vi "Data Change Process.vi"(8 "error in (no error)":errorcluster, 10 "data change":T1={"node ID"="", " value"=variant, "timestamp"=timestamp(0 s since 1904-01-01), "data type"=1, "status code"=0} {"data type" items=["Boolean"=1, "SByte"=2, "Byte"=3, "Int16"=4, "UInt16"=5, "Int32"=6, "UInt32"=7, "Int64"=8, "UInt64"=9, "Float"=10, "Double"=11, "String"=12, "DateTime"=13, "ByteString"=15, "Array of Boolean"=101, "Array of SByte"=102, "Array of Byte"=103, "Array of Int16"=104, "Array of UInt16"=105, "Array of Int32"=106, "Array of UInt32"=107, "Array of Int64"=108, "Array of UInt64"=109, "Array of Float"=110, "Array of Double"=111, "Array of String"=112, "Array of DateTime"=113, "Array of ByteString"=115, "Matrix of Boolean"=201, "Matrix of SByte"=202, "Matrix of Byte"=203, "Matrix of Int16"=204, "Matrix of UInt16"=205, "Matrix of Int32"=206, "Matrix of UInt32"=207, "Matrix of Int64"=208, "Matrix of UInt64"=209, "Matrix of Float"=210, "Matrix of Double"=211, "Matrix of String "=212, "Matrix of DateTime"=213, "Matrix of ByteString"=215]; "status code" items=["Good"=0, "Good_SubscriptionTransferred"=2949120, "Good_CompletesAsynchronously"=3014656, "Good_Overload"=3080192, "Good_Clamped"=3145728, "Good_LocalOverride"=9830400, "Good_EntryInserted"=10616832, "Good_EntryReplaced"=10682368, "Good_NoData"=10813440, "Good_MoreData"=10878976, "Good_CommunicationEvent"=10944512, "Good_ShutdownEvent"=11010048, "Good_CallAgain"=11075584, "Good_NonCriticalTimeout"=11141120, "Good_ResultsMayBeIncomplete"=12189696, "Good_DataIgnored"=14221312, "Uncertain"=1073741824, "Uncertain_ReferenceOutOfServer"=1080819712, "Uncertain_NoCommunicationLastUsableValue"=1083113472, "Uncertain_LastUsableValue"=1083179008, "Uncertain_SubstituteValue"=1083244544, "Uncertain_InitialValue"=1083310080, "Uncertain_SensorNotAccurate"=1083375616, "Uncertain_EngineeringUnitsExceeded"=1083441152, "Uncertain_SubNormal"=1083506688, "Uncertain_DataSubNormal"=1084489728, "Uncertain_ReferenceNotDeleted"=1086062592, "Uncertain_NotAllNodesAvailable"=1086324736, "Bad"=2147483648, "Bad_UnexpectedError"=2147549184, "Bad_InternalError"=2147614720, "Bad_OutOfMemory"=2147680256, "Bad_ResourceUnavailable"=2147745792, "Bad_CommunicationError"=2147811328, "Bad_EncodingError"=2147876864, "Bad_DecodingError"=2147942400, "Bad_EncodingLimitsExceeded"=2148007936, "Bad_UnknownResponse"=2148073472, "Bad_Timeout"=2148139008, "Bad_ServiceUnsupported"=2148204544, "Bad_Shutdown"=2148270080, "Bad_ServerNotConnected"=2148335616, "Bad_ServerHalted"=2148401152, "Bad_NothingToDo"=2148466688, "Bad_TooManyOperations"=2148532224, "Bad_DataTypeIdUnknown"=2148597760, "Bad_CertificateInvalid"=2148663296, "Bad_SecurityChecksFailed"=2148728832, "Bad_CertificateTimeInvalid"=2148794368, "Bad_CertificateIssuerTimeInvalid"=2148859904, "Bad_CertificateHostNameInvalid"=2148925440, "Bad_CertificateUriInvalid"=2148990976, "Bad_CertificateUseNotAllowed"=2149056512, "Bad_CertificateIssuerUseNotAllowed"=2149122048, "Bad_CertificateUntrusted"=2149187584, "Bad_CertificateRevocationUnknown"=2149253120, "Bad_CertificateIssuerRevocationUnknown"=2149318656, "Bad_CertificateRevoked"=2149384192, "Bad_CertificateIssuerRevoked"=2149449728, "Bad_UserAccessDenied"=2149515264, "Bad_IdentityTokenInvalid"=2149580800, "Bad_IdentityTokenRejected"=2149646336, "Bad_SecureChannelIdInvalid"=2149711872, "Bad_InvalidTimestamp"=2149777408, "Bad_NonceInvalid"=2149842944, "Bad_SessionIdInvalid"=2149908480, "Bad_SessionClosed"=2149974016, "Bad_SessionNotActivated"=2150039552, "Bad_SubscriptionIdInvalid"=2150105088, "Bad_RequestHeaderInvalid"=2150236160, "Bad_TimestampsToReturnInvalid"=2150301696, "Bad_RequestCancelledByClient"=2150367232, "Bad_NoCommunication"=2150694912, "Bad_WaitingForInitialData"=2150760448, "Bad_NodeIdInvalid"=2150825984, "Bad_NodeIdUnknown"=2150891520, "Bad_AttributeIdInvalid"=2150957056, "Bad_IndexRangeInvalid"=2151022592, "Bad_IndexRangeNoData"=2151088128, "Bad_DataEncodingInvalid"=2151153664, "Bad_DataEncodingUnsupported"=2151219200, "Bad_NotReadable"=2151284736, "Bad_NotWritable"=2151350272, "Bad_OutOfRange"=2151415808, "Bad_NotSupported"=2151481344, "Bad_NotFound"=2151546880, "Bad_ObjectDeleted"=2151612416, "Bad_NotImplemented"=2151677952, "Bad_MonitoringModeInvalid"=2151743488, "Bad_MonitoredItemIdInvalid"=2151809024, "Bad_MonitoredItemFilterInvalid"=2151874560, "Bad_MonitoredItemFilterUnsupported"=2151940096, "Bad_FilterNotAllowed"=2152005632, "Bad_StructureMissing"=2152071168, "Bad_EventFilterInvalid"=2152136704, "Bad_ContentFilterInvalid"=2152202240, "Bad_FilterOperandInvalid"=2152267776, "Bad_ContinuationPointInvalid"=2152333312, "Bad_NoContinuationPoints"=2152398848, "Bad_ReferenceTypeIdInvalid"=2152464384, "Bad_BrowseDirectionInvalid"=2152529920, "Bad_NodeNotInView"=2152595456, "Bad_ServerUriInvalid"=2152660992, "Bad_ServerNameMissing"=2152726528, "Bad_DiscoveryUrlMissing"=2152792064, "Bad_SempahoreFileMissing"=2152857600, "Bad_RequestTypeInvalid"=2152923136, "Bad_SecurityModeRejected"=2152988672, "Bad_SecurityPolicyRejected"=2153054208, "Bad_TooManySessions"=2153119744, "Bad_UserSignatureInvalid"=2153185280, "Bad_ApplicationSignatureInvalid"=2153250816, "Bad_NoValidCertificates"=2153316352, "Bad_RequestCancelledByRequest"=2153381888, "Bad_ParentNodeIdInvalid"=2153447424, "Bad_ReferenceNotAllowed"=2153512960, "Bad_NodeIdRejected"=2153578496, "Bad_NodeIdExists"=2153644032, "Bad_NodeClassInvalid"=2153709568, "Bad_BrowseNameInvalid"=2153775104, "Bad_BrowseNameDuplicated"=2153840640, "Bad_NodeAttributesInvalid"=2153906176, "Bad_TypeDefinitionInvalid"=2153971712, "Bad_SourceNodeIdInvalid"=2154037248, "Bad_TargetNodeIdInvalid"=2154102784, "Bad_DuplicateReferenceNotAllowed"=2154168320, "Bad_InvalidSelfReference"=2154233856, "Bad_ReferenceLocalOnly"=2154299392, "Bad_NoDeleteRights"=2154364928, "Bad_ServerIndexInvalid"=2154430464, "Bad_ViewIdUnknown"=2154496000, "Bad_TooManyMatches"=2154627072, "Bad_QueryTooComplex"=2154692608, "Bad_NoMatch"=2154758144, "Bad_MaxAgeInvalid"=2154823680, "Bad_HistoryOperationInvalid"=2154889216, "Bad_HistoryOperationUnsupported"=2154954752, "Bad_WriteNotSupported"=2155020288, "Bad_TypeMismatch"=2155085824, "Bad_MethodInvalid"=2155151360, "Bad_ArgumentsMissing"=2155216896, "Bad_TooManySubscriptions"=2155282432, "Bad_TooManyPublishRequests"=2155347968, "Bad_NoSubscription"=2155413504, "Bad_SequenceNumberUnknown"=2155479040, "Bad_MessageNotAvailable"=2155544576, "Bad_InsufficientClientProfile"=2155610112, "Bad_TcpServerTooBusy"=2155675648, "Bad_TcpMessageTypeInvalid"=2155741184, "Bad_TcpSecureChannelUnknown"=2155806720, "Bad_TcpMessageTooLarge"=2155872256, "Bad_TcpNotEnoughResources"=2155937792, "Bad_TcpInternalError"=2156003328, "Bad_TcpEndpointUrlInvalid"=2156068864, "Bad_RequestInterrupted"=2156134400, "Bad_RequestTimeout"=2156199936, "Bad_SecureChannelClosed"=2156265472, "Bad_SecureChannelTokenUnknown"=2156331008, "Bad_SequenceNumberInvalid"=2156396544, "Bad_ConfigurationError"=2156462080, "Bad_NotConnected"=2156527616, "Bad_DeviceFailure"=2156593152, "Bad_SensorFailure"=2156658688, "Bad_OutOfService"=2156724224, "Bad_DeadbandFilterInvalid"=2156789760, "Bad_RefreshInProgress"=2157379584, "Bad_ConditionAlreadyDisabled"=2157445120, "Bad_ConditionDisabled"=2157510656, "Bad_EventIdUnknown"=2157576192, "Bad_NoData"=2157641728, "Bad_DataLost"=2157772800, "Bad_DataUnavailable"=2157838336, "Bad_EntryExists"=2157903872, "Bad_NoEntryExists"=2157969408, "Bad_TimestampNotSupported"=2158034944, "Bad_InvalidArgument"=2158690304, "Bad_ConnectionRejected"=2158755840, "Bad_Disconnect"=2158821376, "Bad_ConnectionClosed"=2158886912, "Bad_InvalidState"=2158952448, "Bad_EndOfStream"=2159017984, "Bad_NoDataAvailable"=2159083520, "Bad_WaitingForResponse"=2159149056, "Bad_OperationAbandoned"=2159214592, "Bad_ExpectedStreamToBlock"=2159280128, "Bad_WouldBlock"=2159345664, "Bad_SyntaxError"=2159411200, "Bad_MaxConnectionsReached"=2159476736, "Bad_RequestTooLarge"=2159542272, "Bad_ResponseTooLarge"=2159607808, "Bad_EventNotAcknowledgeable"=2159738880, "Bad_InvalidTimestampArgument"=2159869952, "Bad_ProtocolVersionUnsupported"=2159935488, "Bad_StateNotActive"=2160001024, "Bad_FilterOperatorInvalid"=2160132096, "Bad_FilterOperatorUnsupported"=2160197632, "Bad_FilterOperandCountMismatch"=2160263168, "Bad_FilterElementInvalid"=2160328704, "Bad_FilterLiteralInvalid"=2160394240, "Bad_IdentityChangeNotSupported"=2160459776, "Bad_NotTypeDefinition"=2160590848, "Bad_ViewTimestampInvalid"=2160656384, "Bad_ViewParameterMismatch"=2160721920, "Bad_ViewVersionInvalid"=2160787456, "Bad_ConditionAlreadyEnabled"=2160852992, "Bad_DialogNotActive"=2160918528, "Bad_DialogResponseInvalid"=2160984064, "Bad_ConditionBranchAlreadyAcked"=2161049600, "Bad_ConditionBranchAlreadyConfirmed"=2161115136, "Bad_ConditionAlreadyShelved"=2161180672, "Bad_ConditionNotShelved"=2161246208, "Bad_ShelvingTimeOutOfRange"=2161311744, "Bad_AggregateListMismatch"=2161377280, "Bad_AggregateNotSupported"=2161442816, "Bad_AggregateInvalidInputs"=2161508352, "Bad_BoundNotFound"=2161573888, "Bad_BoundNotSupported"=2161639424, "Bad_AggregateConfigurationRejected"=2161770496, "Bad_TooManyMonitoredItems"=2161836032]}, 11 "Model in":refnum<class "Model.lvclass">) -> (0 "error out":errorcluster, 3 "Model out":refnum<class "Model.lvclass">)   [LabVIEW 2021, in "Model.lvlib" / "Model.lvclass"]
uses:
  Model.lvclass
  <vilib>/OPCUA/controls/Subscription Data Change.ctl
  <vilib>/OPCUA/controls/NodeId.ctl
  <vilib>/OPCUA/controls/Data Type.ctl
  <vilib>/OPCUA/controls/OPC UA StatusCode.ctl
  Model.lvclass/Model.ctl
  95c299c4-6619-4fcf-af27-bee369d36df4.vi
  <userlib>/John_Lib/AMC_FW/Send Local Message.vi
  <userlib>/John_Lib/AMC_FW/Create Single Message.vi
  <userlib>/John_Lib/AMC_FW/Update Message Routing Info.vi
  <userlib>/John_Lib/OPCUA/add NameSpace for single NoteID.vi
  <vilib>/OPCUA/client/internal/Read.vi
  <vilib>/OPCUA/client/internal/Read String.vi
  <userlib>/John_Lib/AMC_FW/String to Array.vi
  <vilib>/Utility/Data Type/Get Type Information.vi
  <userlib>/John_Lib/AMC_FW/Send Message.vi
  <userlib>/John_Lib/OPCUA/OPCUA.lvclass
  <vilib>/Utility/miscctls.llb/LVStringsAndValuesArrayTypeDef_U16.ctl
panel:
  out "x = y?":bool
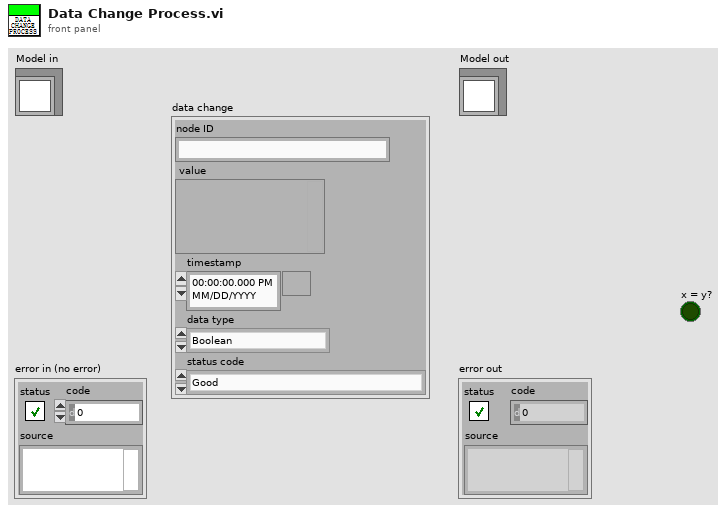
[diagram p1: front panel]
types:
  T1 = typedef "Subscription Data Change.ctl" = cluster{"node ID":T2, " value":variant, "timestamp":timestamp, "data type":T3, "status code":T4}
  T2 = typedef "NodeId.ctl" = string
  T3 = typedef "Data Type.ctl" = u16
  T4 = typedef "OPC UA StatusCode.ctl" = u32
  T5 = typedef "AMC_FW.lvlib/Queue.ctl" = cluster{"Q":T6, "Name":string}
  T6 = typedef "AMC_FW.lvlib/Message Queue.ctl" = refnum<queue>
  T7 = typedef "LVStringsAndValuesArrayTypeDef_U16.ctl" = cluster{"String":string, "Value":u16}[]
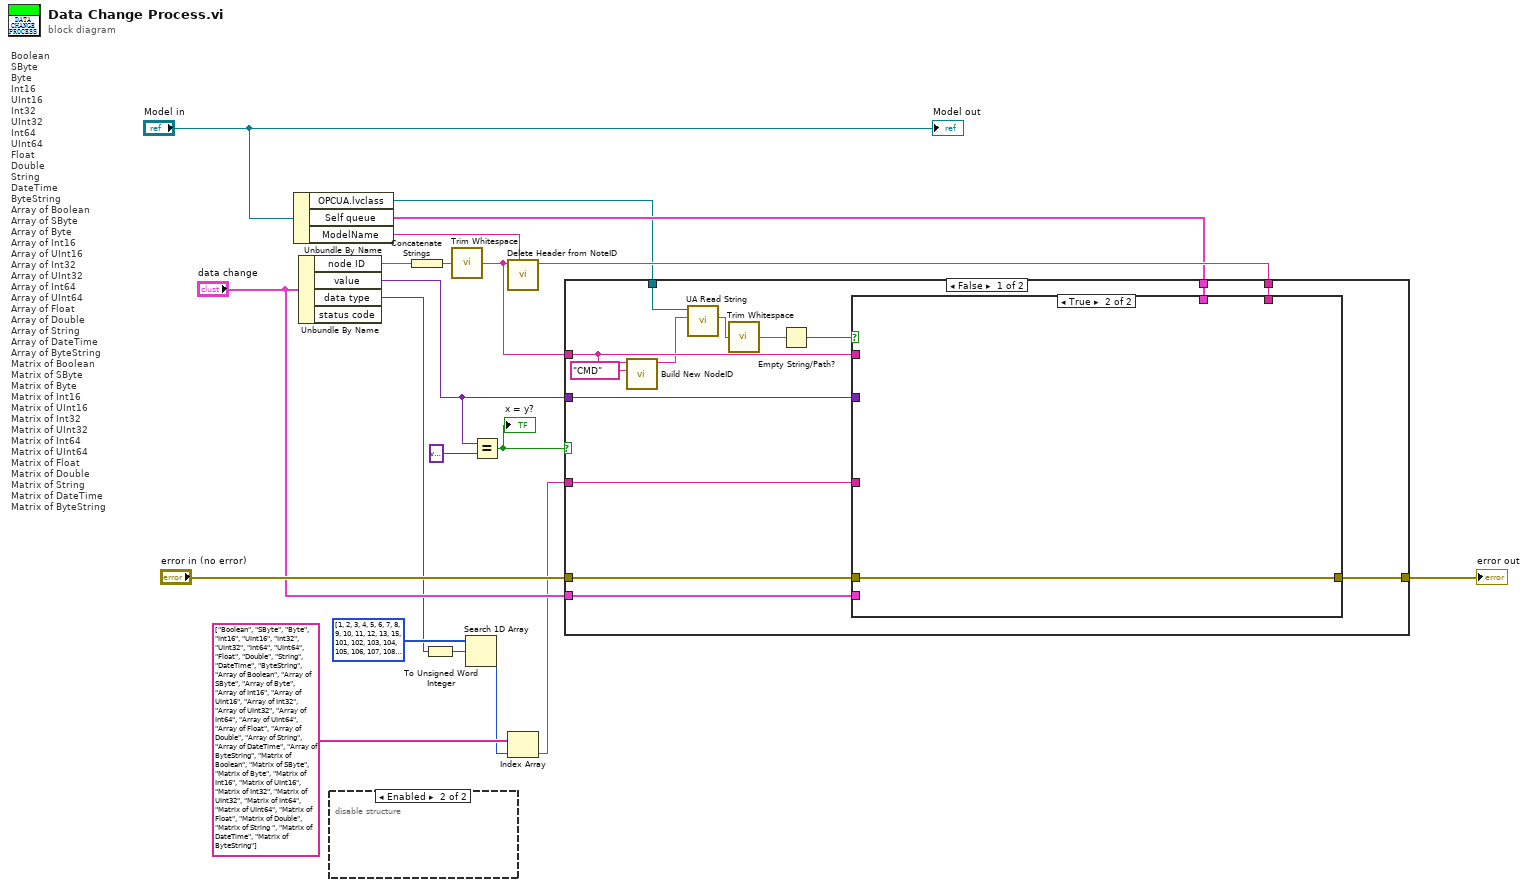
[diagram p0: block diagram]
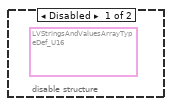
[diagram p2: hidden frame]
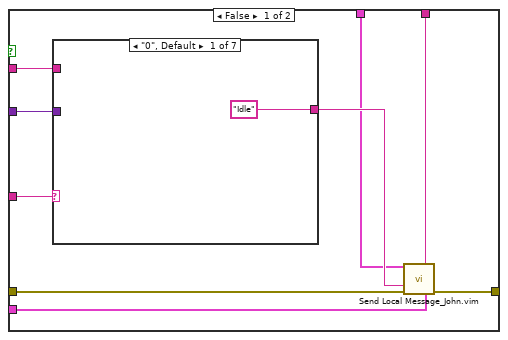
[diagram p3: hidden frame]
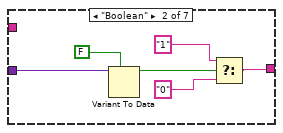
[diagram p4: hidden frame]
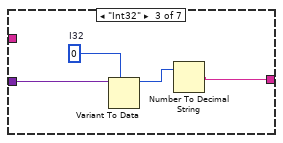
[diagram p5: hidden frame]
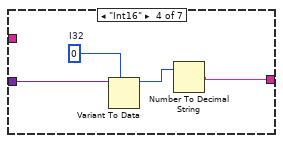
[diagram p6: hidden frame]
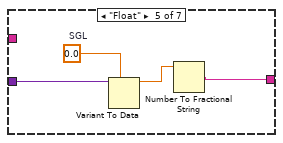
[diagram p7: hidden frame]
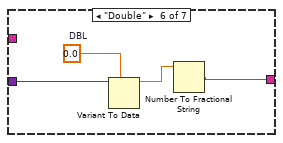
[diagram p8: hidden frame]
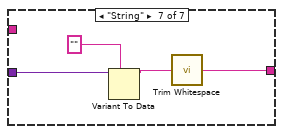
[diagram p9: hidden frame]
diagram:
  # "Boolean\nSByte\nByte\nInt16\nUInt16\nInt32\nUInt32\nInt64\nUInt64\nFloat\nDouble\nString\nDateTime\nByteString\nArray of Boolean\nArray of SByte\nArray of Byte\nArray of Int16\nArray of UInt16\nArray of Int32\nArray of UInt32\nArray of Int64\nArray of UInt64\nArray of Float\nArray of Double\nArray of String\nArray of DateTime\nArray of ByteString\nMatrix of Boolean\nMatrix of SByte\nMatrix of Byte\nMatrix of Int16\nMatrix of UInt16\nMatrix of Int32\nMatrix of UInt32\nMatrix of Int64\nMatrix of UInt64\nMatrix of Float\nMatrix of Double\nMatrix of String \nMatrix of DateTime\nMatrix of ByteString"
  n1 = Unbundle By Name("Model in") -> ("OPCUA.lvclass"=w1:refnum<class "OPCUA.lvclass">, "Self queue"=w14:T5, "ModelName"=w19:string)
  n2 = Unbundle By Name("data change") -> ("node ID"=w18:T2, "value"=w11:variant, "data type"=w6:T3)  [unwired: 1 out]
  n3 = disable-structure shown="Enabled" {
    frame Disabled {
      (unwired) T7 [{"String"="Boolean", "Value"=1}, {"String"="SByte", "Value"=2}, {"String"="Byte", "Value"=3}, {"String"="Int16", "Value"=4}, {"String"="UInt16", "Value"=5}, {"String"="Int32", "Value"=6}, {"String"="UInt32", "Value"=7}, {"String"="Int64", "Value"=8}, {"String"="UInt64", "Value"=9}, {"String"="Float", "Value"=10}, {"String"="Double", "Value"=11}, {"String"="String", "Value"=12}, {"String"="DateTime", "Value"=13}, {"String"="ByteString", "Value"=15}, {"String"="Array of Boolean", "Value"=101}, {"String"="Array of SByte", "Value"=102}, {"String"="Array of Byte", "Value"=103}, {"String"="Array of Int16", "Value"=104}, {"String"="Array of UInt16", "Value"=105}, {"String"="Array of Int32", "Value"=106}, {"String"="Array of UInt32", "Value"=107}, {"String"="Array of Int64", "Value"=108}, {"String"="Array of UInt64", "Value"=109}, {"String"="Array of Float", "Value"=110}, {"String"="Array of Double", "Value"=111}, {"String"="Array of String", "Value"=112}, {"String"="Array of DateTime", "Value"=113}, {"String"="Array of ByteString", "Value"=115}, {"String"="Matrix of Boolean", "Value"=201}, {"String"="Matrix of SByte", "Value"=202}, {"String"="Matrix of Byte", "Value"=203}, {"String"="Matrix of Int16", "Value"=204}, {"String"="Matrix of UInt16", "Value"=205}, {"String"="Matrix of Int32", "Value"=206}, {"String"="Matrix of UInt32", "Value"=207}, {"String"="Matrix of Int64", "Value"=208}, {"String"="Matrix of UInt64", "Value"=209}, {"String"="Matrix of Float", "Value"=210}, {"String"="Matrix of Double", "Value"=211}, {"String"="Matrix of String ", "Value"=212}, {"String"="Matrix of DateTime", "Value"=213}, {"String"="Matrix of ByteString", "Value"=215}] ("Strings And Values []")
    }
    frame Enabled {
    }
  }
  n4 = Concatenate Strings(w18) -> (w17:string)
  n5 = To Unsigned Word Integer(number=w6) -> (unsigned 16bit integer=w5:T3)
  n6 = call <vilib>:"Trim Whitespace.vi"("string"=w17) -> ("trimmed string"=w16:string)  [unwired: 1 in]
  n7 = Search 1D Array(1D array=u16[] [1, 2, 3, 4, 5, 6, 7, 8, 9, 10, 11, 12, 13, 15, 101, 102, 103, 104, 105, 106, 107, 108, 109, 110, 111, 112, 113, 115, 201, 202, 203, 204, 205, 206, 207, 208, 209, 210, 211, 212, 213, 215] ("Array 2"), element=w5) -> (index of element=w3:i32)  [unwired: 1 in]
  n8 = Equal?(x=w11, y=variant ("variant")) -> (x = y?=w9:bool)
  "x = y?" <- w9
  n9 = call <userlib>:"Delete Header from NoteID.vi"("Actor Name"=w19, "node ID full name"=w16) -> ("node ID delete header ns=2;s="=w15:string)  [unwired: 8 in, 1 out]
  n10 = Index Array(array=string[] ["Boolean", "SByte", "Byte", "Int16", "UInt16", "Int32", "UInt32", "Int64", "UInt64", "Float", "Double", "String", "DateTime", "ByteString", "Array of Boolean", "Array of SByte", "Array of Byte", "Array of Int16", "Array of UInt16", "Array of Int32", "Array of UInt32", "Array of Int64", "Array of UInt64", "Array of Float", "Array of Double", "Array of String", "Array of DateTime", "Array of ByteString", "Matrix of Boolean", "Matrix of SByte", "Matrix of Byte", "Matrix of Int16", "Matrix of UInt16", "Matrix of Int32", "Matrix of UInt32", "Matrix of Int64", "Matrix of UInt64", "Matrix of Float", "Matrix of Double", "Matrix of String ", "Matrix of DateTime", "Matrix of ByteString"] ("Array"), index=w3) -> (element=w2:string)
  n11 = case shown="False" w9 {
    tunnel: w2 -> [w34 _]
    tunnel: w16 -> [w26 _]
    tunnel: w15 -> [w33 _]
    tunnel: w14 -> [w32 _]
    tunnel: "error in (no error)" -> [w31 w72]
    tunnel: [w30 w72] -> w12
    tunnel: w11 -> [w29 _]
    tunnel: "data change" -> [w28 _]
    tunnel: w1 -> [w27 _]
    frame False {
      n12 = call <userlib>:"Build New NodeID.vi"("SubName"="CMD", "node ID"=w26) -> ("concatenated string"=w24:string)  [unwired: 6 in, 3 out]
      n13 = call <userlib>:"UA Read String.vi"("node ID"=w24, "OPCUA in"=w27) -> ("value"=w23:string)  [unwired: 5 in, 4 out]
      n14 = call <vilib>:"Trim Whitespace.vi"("string"=w23) -> ("trimmed string"=w22:string)  [unwired: 1 in]
      n15 = Empty String/Path?(string/path=w22) -> (empty?=w21:bool)
      n16 = case shown="True" w21 {
        tunnel: w34 -> [w43 _]
        tunnel: w33 -> [w41 _]
        tunnel: w32 -> [w40 _]
        tunnel: w31 -> [w39 w71]
        tunnel: [w38 w71] -> w30
        tunnel: w29 -> [w37 _]
        tunnel: w28 -> [w36 _]
        tunnel: w26 -> [w35 _]
        frame False {
          n17 = case shown="\"0\", Default" w43 {
            tunnel: w37 -> [_ w50 w54 w58 w62 w66 w70]
            tunnel: w35 -> [_ _ _ _ _ _ _]
            tunnel: ["Idle" ("DBL") w45 w51 w55 w59 w63 w67] -> w42
            frame "0", Default {
            }
            frame "Boolean" {
              n18 = Variant To Data(type=FALSE, Variant=w50) -> (data=w48:bool)  [unwired: 1 in, 1 out]
              n19 = Select(t="1" ("ModelName"), s=w48, f="0") -> (s? t:f=w45:string)
            }
            frame "Int32" {
              w53 = 0  # I32
              n20 = Variant To Data(type=w53, Variant=w54) -> (data=w52:i32)  [unwired: 1 in, 1 out]
              n21 = Number To Decimal String(number=w52) -> (decimal integer string=w51:string)  [unwired: 1 in]
            }
            frame "Int16" {
              w57 = i16 0  # I32
              n22 = Variant To Data(type=w57, Variant=w58) -> (data=w56:i16)  [unwired: 1 in, 1 out]
              n23 = Number To Decimal String(number=w56) -> (decimal integer string=w55:string)  [unwired: 1 in]
            }
            frame "Float" {
              w61 = sgl 0.0  # SGL
              n24 = Variant To Data(type=w61, Variant=w62) -> (data=w60:sgl)  [unwired: 1 in, 1 out]
              n25 = Number To Fractional String(number=w60) -> (F-format string=w59:string)  [unwired: 3 in]
            }
            frame "Double" {
              w65 = 0.0  # DBL
              n26 = Variant To Data(type=w65, Variant=w66) -> (data=w64:dbl)  [unwired: 1 in, 1 out]
              n27 = Number To Fractional String(number=w64) -> (F-format string=w63:string)  [unwired: 3 in]
            }
            frame "String" {
              n28 = Variant To Data(type="" ("DBL"), Variant=w70) -> (data=w68:string)  [unwired: 1 in, 1 out]
              n29 = call <vilib>:"Trim Whitespace.vi"("string"=w68) -> ("trimmed string"=w67:string)  [unwired: 1 in]
            }
          }
          n30 = call "Send Local Message_John.vim"("Queue In"=w40, "Elements in Front"=w41, "message value"=w42, "error in"=w39, "variant"=w36) -> ("error out"=w38:errorcluster)  [unwired: 8 in, 2 out]
        }
        frame True {
        }
      }
    }
    frame True {
    }
  }
  "error out" <- w12
  "Model out" <- "Model in"
